vi "SetInTriggerMode.vi"(6 "Delay between send and receive [ms]":i32=100, 8 "error in (no error)":errorcluster, 10 "mode":i32, 11 "SCD in":refnum<class "SCD.lvclass">) -> (0 "error out":errorcluster, 3 "SCD out":refnum<class "SCD.lvclass">)   [LabVIEW 2020, in "horiba.lvlib" / "SCD.lvclass"]
doc: "Tell the device how Hardware Trigger pin is used. Returns Error if Acquisition is in Progress.\n\nmode: Mode of hardware trigger pin.\n0: TTL input\n1: Event marker input\n2: Hardware trigger input"
uses:
  SCD.lvclass
  SCD.lvclass/SCD.ctl
  b6349250-cb33-415b-847a-a7f5d99734f6.vi
  GenericDevice/GenericDevice.lvclass
  ca73f763-8e2b-4d84-8e4e-0e6044455bd1.vi
panel:
  # "Connector Pane"
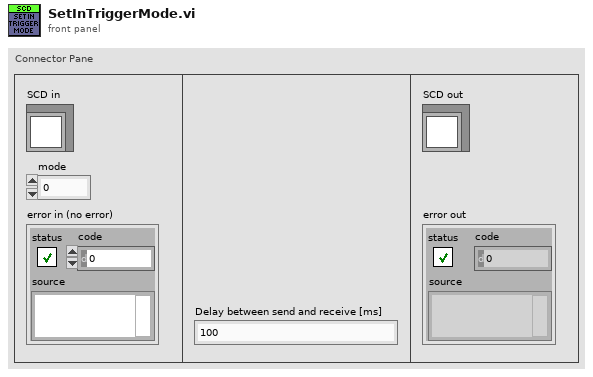
[diagram p1: front panel]
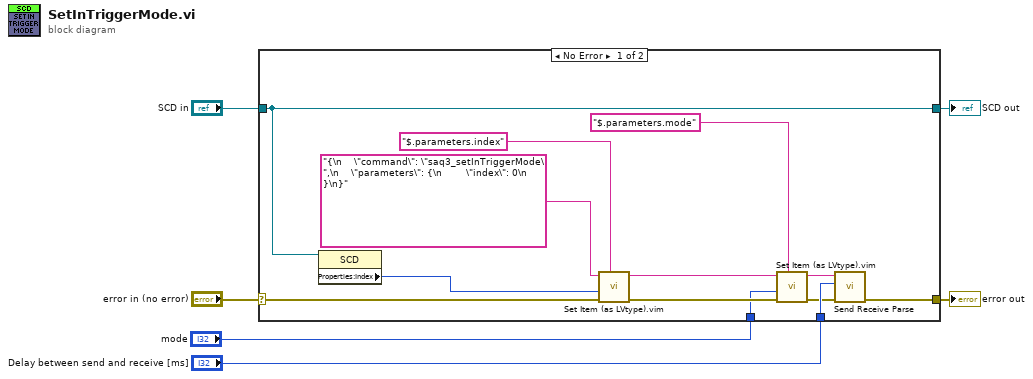
[diagram p0: block diagram]
diagram:
  n1 = case shown="No Error" "error in (no error)" {
    selector: "error in (no error)" -> [w15 w21]
    tunnel: [w13 w21] -> w2
    tunnel: [w17 w20] -> w4
    tunnel: "SCD in" -> [w17 w20]
    tunnel: "Delay between send and receive [ms]" -> [w12 _]
    tunnel: "mode" -> [w7 _]
    frame No Error {
      n2 = property class="SCD"(reference=w17) -> ("Properties:Index"=w16:i32)  [unwired: 1 in, 2 out]
      n3 = call "Set Item (as LVtype).vim"("$Path or Item Name"="$.parameters.index", "error in (no error)"=w15, "Anything"=w16, "JSON"="{\n    \"command\": \"saq3_setInTriggerMode\",\n    \"parameters\": {\n        \"index\": 0\n    }\n}") -> ("error out"=w14:errorcluster, "<JSON>"=w10:string)  [unwired: 4 in, 1 out]
      n4 = call "Set Item (as LVtype).vim"("$Path or Item Name"="$.parameters.mode", "error in (no error)"=w14, "Anything"=w7, "JSON"=w10) -> ("error out"=w11:errorcluster, "<JSON>"=w9:string)  [unwired: 4 in, 1 out]
      n5 = call "Send Receive Parse.vi"("error in"=w11, "Delay between send and receive [ms]"=w12, "<JSON>"=w9) -> ("error out"=w13:errorcluster)  [unwired: 6 in, 2 out]
    }
    frame Error {
    }
  }
  "error out" <- w2
  "SCD out" <- w4
